vi "G_code_interpriter.vi"() -> ()   [LabVIEW 2019]
uses:
  <vilib>/Instr/_visa.llb/VISA Configure Serial Port (Instr).vi
panel:
  in  "Выберите COM порт, к которому\nподключено устрйоство":refnum<visa-resource-name>
  in  "stop":bool
  in  "Выбор режима":enum32{"Автоматический режи", "Ручной режим"}(tab)
  out "Номер выполняемой\nстроки":i32
  out "Сейчас выполняется":string[](array[string])
  in  "Исполняемый код":string="%\nG00 X50 Y50 Z10\nG01 X80 Y80\nG03 X120 Y120\nG04 P500\nG03 X50 Y50\nG00 X50 Y50 Z50\nM30\n"
  in  "Автоматический режим старт":bool
  in  "Вверх 2":bool
  in  "?":T1(radio)
  in  "Вниз 2":bool
  in  "Ручной режим старт":bool
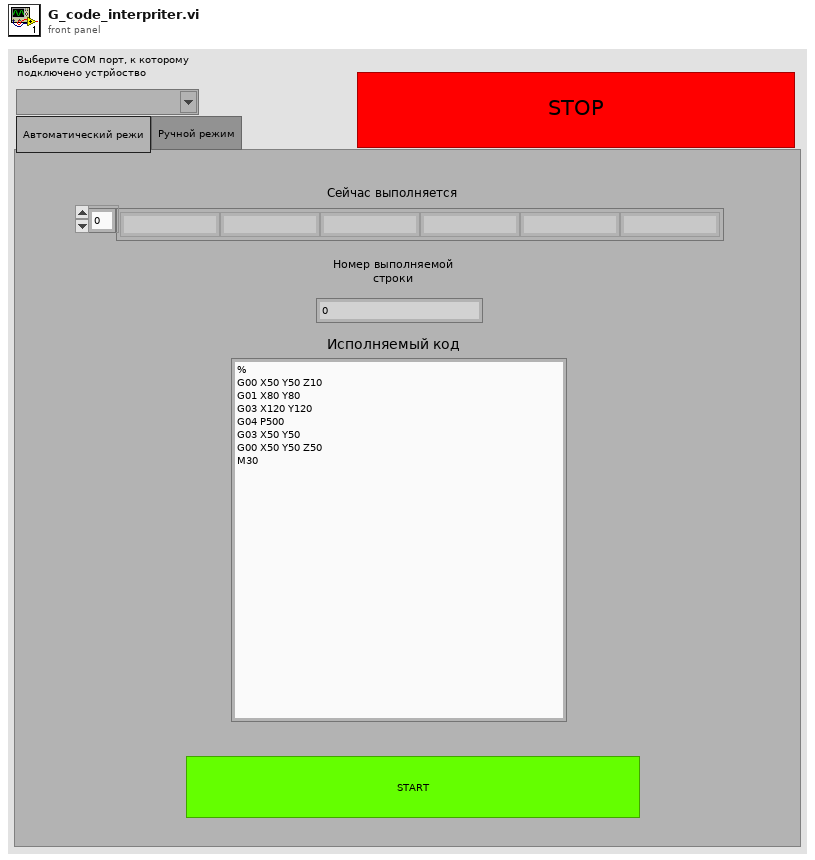
[diagram p1: front panel]
types:
  T1 = enum32{"Перемещение по координате X, 1мм", "Перемещение по координате Y, 1мм", "Перемещение по координате Z, 1мм", "Вращение схвата"}
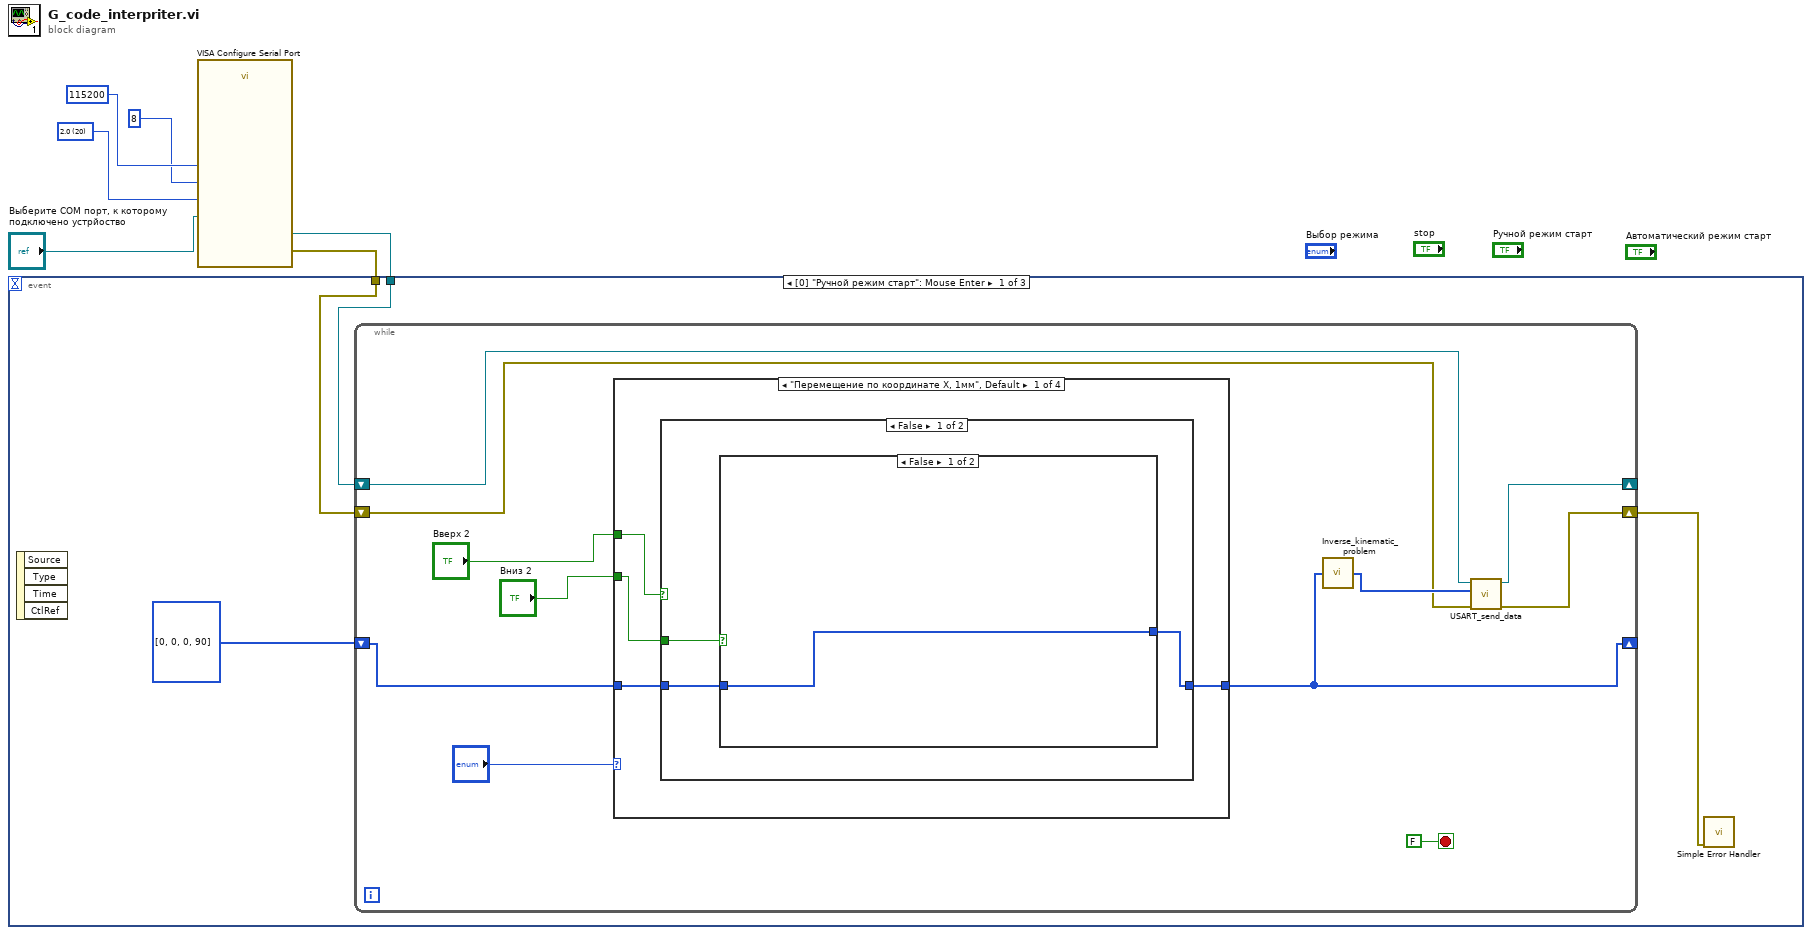
[diagram p0: block diagram]
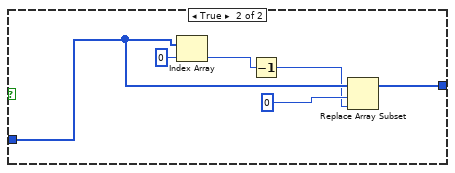
[diagram p2: hidden frame]
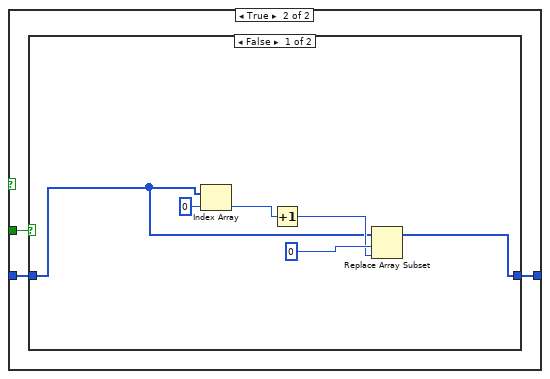
[diagram p3: hidden frame]
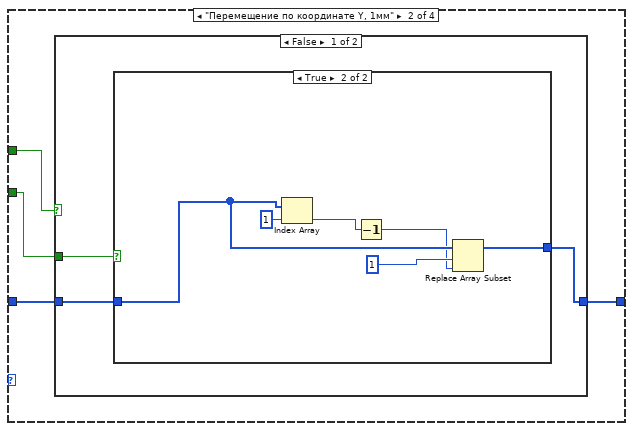
[diagram p5: hidden frame]
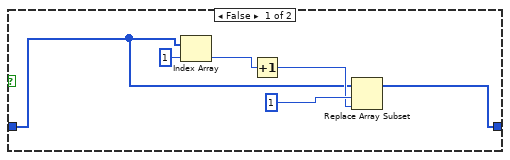
[diagram p8: hidden frame]
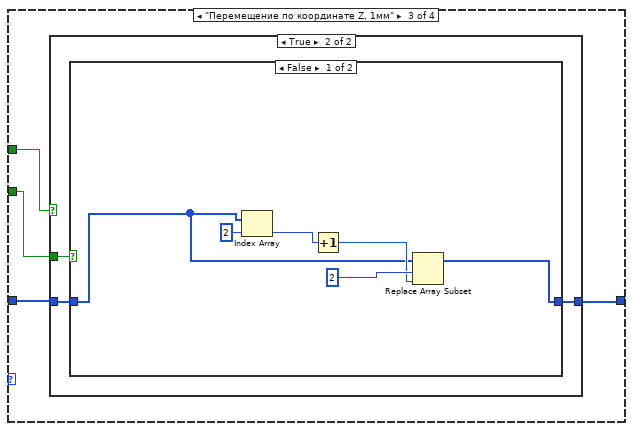
[diagram p9: hidden frame]
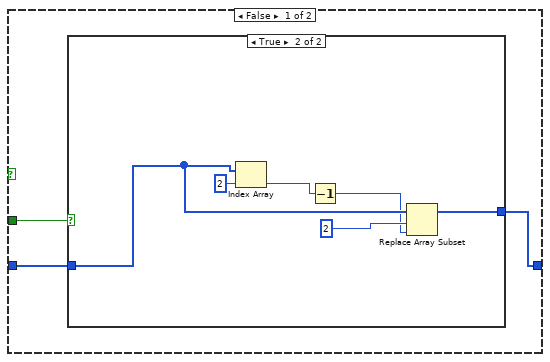
[diagram p10: hidden frame]
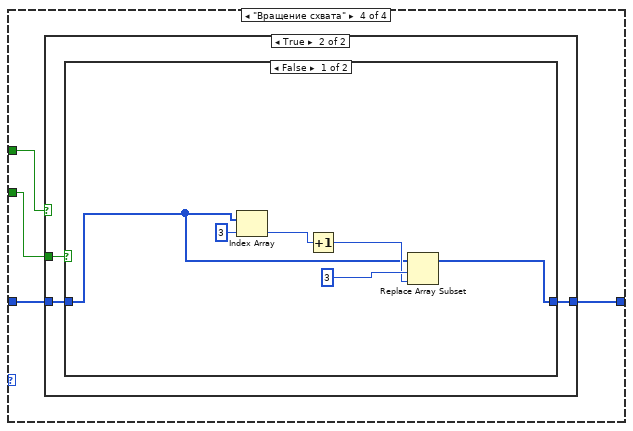
[diagram p13: hidden frame]
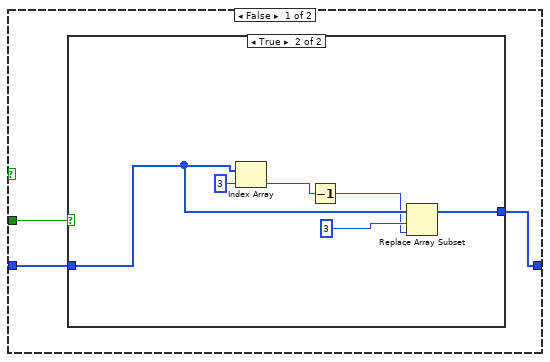
[diagram p14: hidden frame]
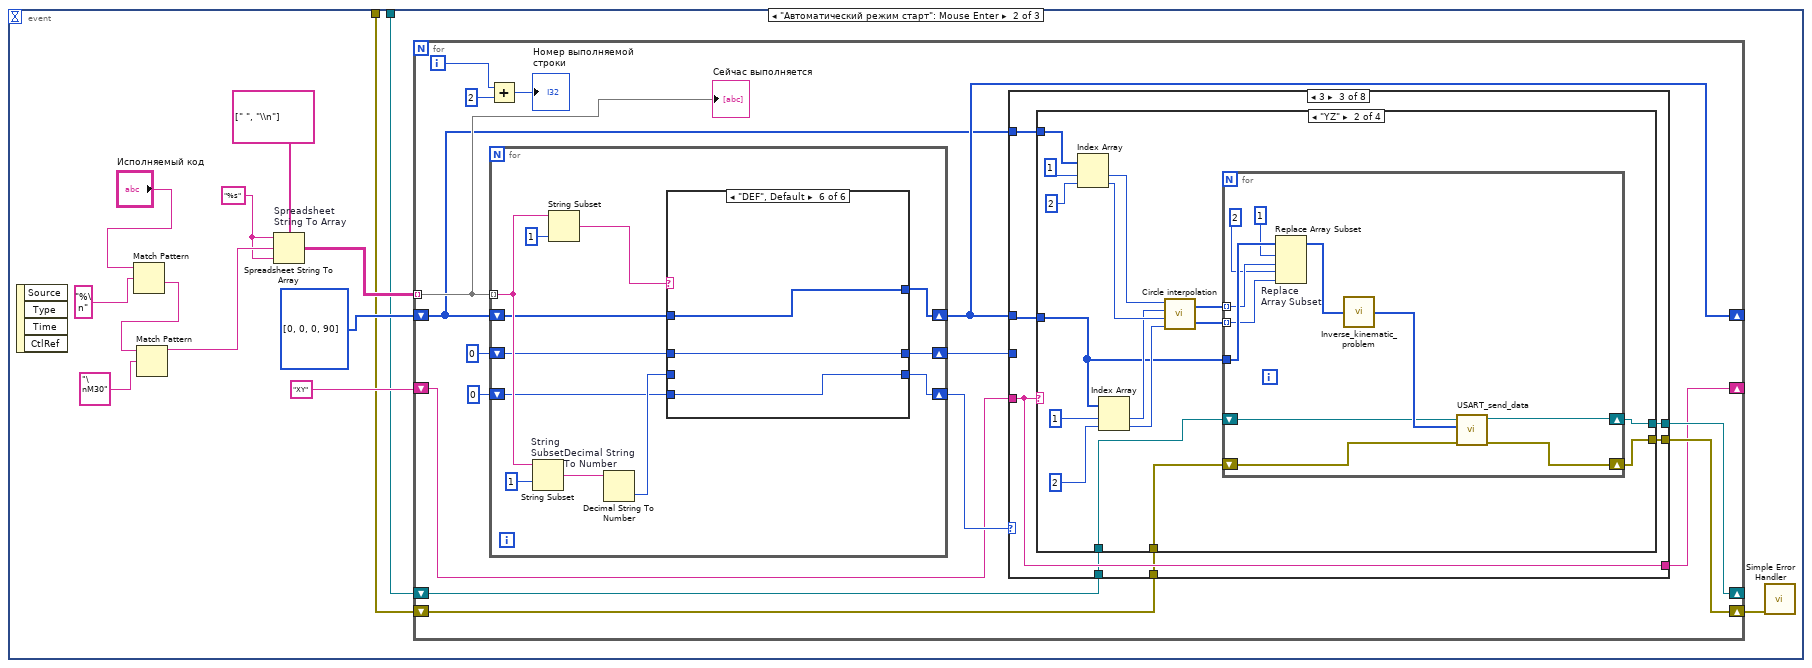
[diagram p17: hidden frame]
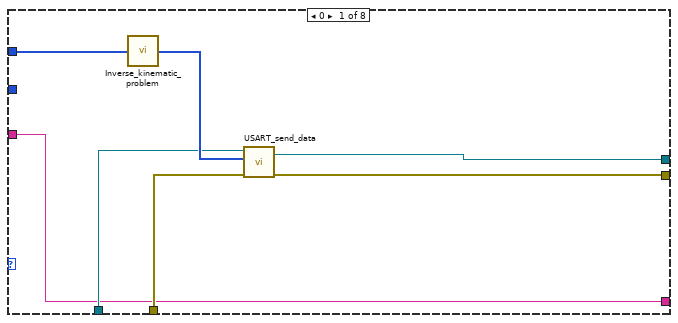
[diagram p18: hidden frame]
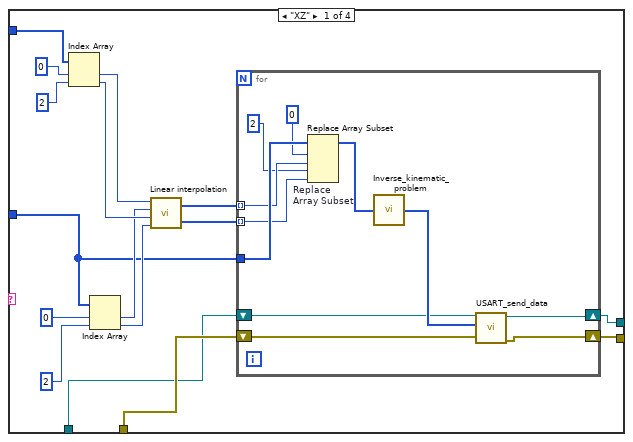
[diagram p20: hidden frame]
diagram:
  w3 = u16 20 items=["1.0"=10, "1.5"=15, "2.0"=20] ("stop bits (10: 1 bit)")
  n1 = call-poly "VISA Configure Serial Port"("VISA resource name"="Выберите COM порт, к которому\nподключено устрйоство", "baud rate (9600)"=u32 115200, "data bits (8)"=u16 8, "stop bits (10: 1 bit)"=w3) -> ("VISA resource name out"=w1:refnum<visa-resource-name>, "error out"=w2:errorcluster)  [unwired: 10 in]
  n2 = event shown="[0] \"Ручной режим старт\": Mouse Enter" {
    selector: _ -> [_ _ _]
    dyn-events: _ -> [_ _ _]
    timeout: _ -> [_ _ _]
    tunnel: w1 -> [w9 w119 _]
    tunnel: w2 -> [w8 w118 _]
    event "Ручной режим старт": Mouse Enter {
      n3 = event-data() -> ()  [unwired: 1 in, 4 out]
      n4 = while {
        shift-right: [w11] -> _
        shift-left: i32[] [0, 0, 0, 90] -> [w18]
        shift-right: [w13] -> _
        shift-left: w9 -> [w15]
        shift-right: [w12] -> w7
        shift-left: w8 -> [w14]
        stop <- FALSE stop-if-true
        n5 = case shown="\"Перемещение по координате X, 1мм\", Default" "?" {
          tunnel: w18 -> [w23 w49 w73 w97]
          tunnel: "Вверх 2" -> [w25 w48 w71 w95]
          tunnel: "Вниз 2" -> [w24 w47 w70 w94]
          tunnel: [w22 w46 w72 w96] -> w11
          frame "Перемещение по координате X, 1мм", Default {
            n6 = case shown="False" w25 {
              tunnel: w24 -> [w28 w38]
              tunnel: w23 -> [w27 w37]
              tunnel: [w26 w36] -> w22
              frame False {
                n7 = case shown="False" w28 {
                  tunnel: w27 -> [w29 w33]
                  tunnel: [w29 w30] -> w26
                  frame False {
                  }
                  frame True {
                    n8 = Index Array(array=w33, index=0) -> (element=w31:i32)
                    n9 = Decrement(x=w31) -> (x-1=w32:i32)
                    n10 = Replace Array Subset(array=w33, new element=w32, index=0) -> (w30:i32[])
                  }
                }
              }
              frame True {
                n11 = case shown="False" w38 {
                  tunnel: w37 -> [w40 w45]
                  tunnel: [w39 w45] -> w36
                  frame False {
                    n12 = Index Array(array=w40, index=0) -> (element=w43:i32)
                    n13 = Increment(x=w43) -> (x+1=w41:i32)
                    n14 = Replace Array Subset(array=w40, new element=w41, index=0) -> (w39:i32[])
                  }
                  frame True {
                  }
                }
              }
            }
          }
          frame "Перемещение по координате Y, 1мм" {
            n15 = case shown="False" w48 {
              tunnel: w47 -> [w52 w62]
              tunnel: w49 -> [w51 w61]
              tunnel: [w50 w60] -> w46
              frame False {
                n16 = case shown="True" w52 {
                  tunnel: w51 -> [w53 w57]
                  tunnel: [w53 w54] -> w50
                  frame False {
                  }
                  frame True {
                    n17 = Index Array(array=w57, index=1) -> (element=w55:i32)
                    n18 = Decrement(x=w55) -> (x-1=w56:i32)
                    n19 = Replace Array Subset(array=w57, new element=w56, index=1) -> (w54:i32[])
                  }
                }
              }
              frame True {
                n20 = case shown="True" w62 {
                  tunnel: w61 -> [w64 w69]
                  tunnel: [w63 w69] -> w60
                  frame False {
                    n21 = Index Array(array=w64, index=1) -> (element=w67:i32)
                    n22 = Increment(x=w67) -> (x+1=w65:i32)
                    n23 = Replace Array Subset(array=w64, new element=w65, index=1) -> (w63:i32[])
                  }
                  frame True {
                  }
                }
              }
            }
          }
          frame "Перемещение по координате Z, 1мм" {
            n24 = case shown="True" w71 {
              tunnel: w70 -> [w76 w86]
              tunnel: w73 -> [w75 w85]
              tunnel: [w74 w84] -> w72
              frame False {
                n25 = case shown="True" w76 {
                  tunnel: w75 -> [w77 w81]
                  tunnel: [w77 w78] -> w74
                  frame False {
                  }
                  frame True {
                    n26 = Index Array(array=w81, index=2) -> (element=w79:i32)
                    n27 = Decrement(x=w79) -> (x-1=w80:i32)
                    n28 = Replace Array Subset(array=w81, new element=w80, index=2) -> (w78:i32[])
                  }
                }
              }
              frame True {
                n29 = case shown="False" w86 {
                  tunnel: w85 -> [w88 w93]
                  tunnel: [w87 w93] -> w84
                  frame False {
                    n30 = Index Array(array=w88, index=2) -> (element=w91:i32)
                    n31 = Increment(x=w91) -> (x+1=w89:i32)
                    n32 = Replace Array Subset(array=w88, new element=w89, index=2) -> (w87:i32[])
                  }
                  frame True {
                  }
                }
              }
            }
          }
          frame "Вращение схвата" {
            n33 = case shown="True" w95 {
              tunnel: w94 -> [w100 w110]
              tunnel: w97 -> [w99 w109]
              tunnel: [w98 w108] -> w96
              frame False {
                n34 = case shown="True" w100 {
                  tunnel: w99 -> [w101 w105]
                  tunnel: [w101 w102] -> w98
                  frame False {
                  }
                  frame True {
                    n35 = Index Array(array=w105, index=3) -> (element=w103:i32)
                    n36 = Decrement(x=w103) -> (x-1=w104:i32)
                    n37 = Replace Array Subset(array=w105, new element=w104, index=3) -> (w102:i32[])
                  }
                }
              }
              frame True {
                n38 = case shown="False" w110 {
                  tunnel: w109 -> [w112 w117]
                  tunnel: [w111 w117] -> w108
                  frame False {
                    n39 = Index Array(array=w112, index=3) -> (element=w115:i32)
                    n40 = Increment(x=w115) -> (x+1=w113:i32)
                    n41 = Replace Array Subset(array=w112, new element=w113, index=3) -> (w111:i32[])
                  }
                  frame True {
                  }
                }
              }
            }
          }
        }
        n42 = call "Inverse_kinematic_problem.vi"("Необходимое\nположение\nсхвата"=w11) -> ("Coords"=w16:u32[])
        n43 = call "USART_send_data.vi"("error in"=w14, "Coordinates"=w16, "VISA resource name in"=w15) -> ("error out"=w12:errorcluster, "VISA resource name out"=w13:refnum<visa-resource-name>)  [unwired: 7 in]
      }
      n44 = call <vilib>:"Simple Error Handler.vi"("error in (no error)"=w7) -> ()  [unwired: 4 in, 5 out]
    }
    event "Автоматический режим старт": Mouse Enter {
      w121 = "%s" ("format string")
      n45 = event-data() -> ()  [unwired: 1 in, 4 out]
      n46 = Match Pattern(string="Исполняемый код", regular expression="%\n") -> (after substring=w126:string)  [unwired: 1 in, 3 out]
      n47 = Match Pattern(string=w126, regular expression="\nM30") -> (before substring=w127:string)  [unwired: 1 in, 3 out]
      n48 = Spreadsheet String To Array "Spreadsheet\nString To Array"(delimiter (Tab)=string[] [" ", "\\n"], format string=w121, spreadsheet string=w127, array type (2D Dbl)=w121) -> (array=w128:string[][])
      n49 = for {
        tunnel: w128 -> [w146] mode=indexing
        shift-right: [w141] -> _
        shift-left: i32[] [0, 0, 0, 90] -> [w140]
        shift-right: [w139] -> w129
        shift-left: w118 -> [w138]
        shift-right: [w134] -> _
        shift-left: "XY" -> [w137]
        shift-right: [w135] -> _
        shift-left: w119 -> [w136]
        i -> [w133]
        n50 = Add(x=w133, y=2) -> (x+y=→"Номер выполняемой\nстроки":i32)
        n51 = for {
          tunnel: w146 -> [w366] mode=indexing
          shift-right: [w357] -> w143
          shift-left: 0 -> [w360]
          shift-right: [w358] -> w141
          shift-left: w140 -> [w359]
          shift-right: [w356] -> w142
          shift-left: 0 -> [w355]
          n52 = String Subset "String\nSubset"(string=w366, offset (0)=1) -> (substring=w362:string)  [unwired: 1 in]
          n53 = String Subset(string=w366, length (rest)=1 ("length (rest)")) -> (substring=w363:string)  [unwired: 1 in]
          n54 = Decimal String To Number "Decimal String\nTo Number"(string=w362) -> (number=w361:i32)  [unwired: 2 in, 1 out]
          n55 = case shown="\"DEF\", Default" w363 {
            tunnel: w361 -> [w369 w373 w379 w385 w388 _]
            tunnel: [w369 w375 w381 w387 w389 w393] -> w357
            tunnel: w360 -> [_ w375 w381 w387 w389 w393]
            tunnel: w359 -> [w368 w374 w378 w384 w390 w392]
            tunnel: [w368 w371 w377 w383 w390 w392] -> w358
            tunnel: [w367 w370 w376 w382 w388 w391] -> w356
            tunnel: w355 -> [w367 w370 w376 w382 _ w391]
            frame "G" {
            }
            frame "X" {
              n56 = Replace Array Subset(array=w374, new element=w373, index=0) -> (w371:i32[])
            }
            frame "Y" {
              n57 = Replace Array Subset(array=w378, new element=w379, index=1) -> (w377:i32[])
            }
            frame "Z" {
              n58 = Replace Array Subset "Replace Array Subset"(array=w384, new element=w385, index=2) -> (w383:i32[])
            }
            frame "P" {
            }
            frame "DEF", Default {
            }
          }
        }
        n59 = case shown="3" w143 {
          tunnel: w142 -> [_ _ _ w337 _ _ _ _]
          tunnel: w141 -> [w153 w159 w249 _ _ _ _ _]
          tunnel: w140 -> [_ w160 w248 _ _ _ _ _]
          tunnel: w136 -> [w151 w157 w246 w335 w339 w342 w345 w348]
          tunnel: w138 -> [w150 w158 w247 w336 w340 w343 w346 w349]
          tunnel: [w149 w156 w244 w336 w340 w343 w346 w349] -> w139
          tunnel: w137 -> [w147 w154 w250 w334 _ _ _ w347]
          tunnel: [w148 w155 w245 w335 w339 w342 w345 w348] -> w135
          tunnel: [w147 w154 w250 w334 "XY" "XZ" "YZ" w347] -> w134
          frame 0 {
            n60 = call "Inverse_kinematic_problem.vi"("Необходимое\nположение\nсхвата"=w153) -> ("Coords"=w152:u32[])
            n61 = call "USART_send_data.vi"("error in"=w150, "Coordinates"=w152, "VISA resource name in"=w151) -> ("error out"=w149:errorcluster, "VISA resource name out"=w148:refnum<visa-resource-name>)  [unwired: 7 in]
          }
          frame 1 {
            n62 = case shown="\"DEF\", Default" w154 {
              tunnel: w160 -> [w166 w193 w220 _]
              tunnel: w159 -> [w165 w192 w218 _]
              tunnel: w158 -> [w164 w191 w219 w243]
              tunnel: w157 -> [w162 w189 w216 w242]
              tunnel: [w163 w190 w217 w243] -> w156
              tunnel: [w161 w188 w215 w242] -> w155
              frame "XZ" {
                n63 = Index Array(array=w166, index #1=0 ("index"), index #2=2 ("index")) -> (element #1=w172:i32, element #2=w171:i32)
                n64 = Index Array(array=w165, index #1=0 ("index"), index #2=2 ("index")) -> (element #1=w170:i32, element #2=w169:i32)
                n65 = call "Linear interpolation.vi"("Yf"=w169, "Y0"=w171, "Xf"=w170, "X0"=w172) -> ("Y array"=w167:i32[], "X array"=w168:i32[])
                n66 = for {
                  tunnel: w168 -> [w186] mode=indexing
                  tunnel: w167 -> [w185] mode=indexing
                  tunnel: w165 -> [w187]
                  shift-right: [w179] -> w163
                  shift-left: w164 -> [w180]
                  shift-right: [w177] -> w161
                  shift-left: w162 -> [w178]
                  n67 = Replace Array Subset "Replace\nArray Subset"(array=w187, new element #1=w186, index #1=0 ("index"), new element #2=w185, index #2=2 ("index")) -> (w181:i32[])
                  n68 = call "Inverse_kinematic_problem.vi"("Необходимое\nположение\nсхвата"=w181) -> ("Coords"=w182:u32[])
                  n69 = call "USART_send_data.vi"("error in"=w180, "Coordinates"=w182, "VISA resource name in"=w178) -> ("error out"=w179:errorcluster, "VISA resource name out"=w177:refnum<visa-resource-name>)  [unwired: 7 in]
                }
              }
              frame "XY" {
                n70 = Index Array(array=w193, index #1=0 ("index"), index #2=1 ("index")) -> (element #1=w199:i32, element #2=w198:i32)
                n71 = Index Array(array=w192, index #1=0 ("index"), index #2=1 ("index")) -> (element #1=w197:i32, element #2=w196:i32)
                n72 = call "Linear interpolation.vi"("Yf"=w196, "Y0"=w198, "Xf"=w197, "X0"=w199) -> ("Y array"=w194:i32[], "X array"=w195:i32[])
                n73 = for {
                  tunnel: w195 -> [w213] mode=indexing
                  tunnel: w194 -> [w212] mode=indexing
                  tunnel: w192 -> [w214]
                  shift-right: [w206] -> w190
                  shift-left: w191 -> [w207]
                  shift-right: [w204] -> w188
                  shift-left: w189 -> [w205]
                  n74 = Replace Array Subset "Replace\nArray Subset"(array=w214, new element #1=w213, index #1=0 ("index"), new element #2=w212, index #2=1 ("index")) -> (w208:i32[])
                  n75 = call "Inverse_kinematic_problem.vi"("Необходимое\nположение\nсхвата"=w208) -> ("Coords"=w209:u32[])
                  n76 = call "USART_send_data.vi"("error in"=w207, "Coordinates"=w209, "VISA resource name in"=w205) -> ("error out"=w206:errorcluster, "VISA resource name out"=w204:refnum<visa-resource-name>)  [unwired: 7 in]
                }
              }
              frame "YZ" {
                n77 = Index Array(array=w220, index #1=1 ("index"), index #2=2 ("index")) -> (element #1=w226:i32, element #2=w225:i32)
                n78 = Index Array(array=w218, index #1=1 ("index"), index #2=2 ("index")) -> (element #1=w224:i32, element #2=w223:i32)
                n79 = call "Linear interpolation.vi"("Yf"=w223, "Y0"=w225, "Xf"=w224, "X0"=w226) -> ("Y array"=w221:i32[], "X array"=w222:i32[])
                n80 = for {
                  tunnel: w222 -> [w240] mode=indexing
                  tunnel: w221 -> [w239] mode=indexing
                  tunnel: w218 -> [w241]
                  shift-right: [w233] -> w217
                  shift-left: w219 -> [w234]
                  shift-right: [w231] -> w215
                  shift-left: w216 -> [w232]
                  n81 = Replace Array Subset "Replace\nArray Subset"(array=w241, new element #1=w240, index #1=1 ("index"), new element #2=w239, index #2=2 ("index")) -> (w235:i32[])
                  n82 = call "Inverse_kinematic_problem.vi"("Необходимое\nположение\nсхвата"=w235) -> ("Coords"=w236:u32[])
                  n83 = call "USART_send_data.vi"("error in"=w234, "Coordinates"=w236, "VISA resource name in"=w232) -> ("error out"=w233:errorcluster, "VISA resource name out"=w231:refnum<visa-resource-name>)  [unwired: 7 in]
                }
              }
              frame "DEF", Default {
              }
            }
          }
          frame 3 {
            n84 = case shown="\"YZ\"" w250 {
              tunnel: w249 -> [w255 w283 _ w312]
              tunnel: w248 -> [w256 w282 _ w311]
              tunnel: w247 -> [w253 w280 w305 w310]
              tunnel: w246 -> [w254 w281 w306 w309]
              tunnel: [w252 w279 w306 w308] -> w245
              tunnel: [w251 w278 w305 w307] -> w244
              frame "XZ" {
                n85 = Index Array(array=w256, index #1=0 ("index"), index #2=2 ("index")) -> (element #1=w261:i32, element #2=w263:i32)
                n86 = Index Array(array=w255, index #1=0 ("index"), index #2=2 ("index")) -> (element #1=w262:i32, element #2=w264:i32)
                n87 = call "Circle interpolation.vi"("Yf"=w264, "Y0"=w263, "Xf"=w262, "X0"=w261) -> ("Y array"=w265:i32[], "X array"=w266:i32[])
                n88 = for {
                  tunnel: w266 -> [w276] mode=indexing
                  tunnel: w265 -> [w275] mode=indexing
                  tunnel: w255 -> [w277]
                  shift-right: [w269] -> w251
                  shift-left: w253 -> [w270]
                  shift-right: [w267] -> w252
                  shift-left: w254 -> [w268]
                  n89 = Replace Array Subset "Replace\nArray Subset"(array=w277, new element #1=w276, index #1=0 ("index"), new element #2=w275, index #2=2 ("index")) -> (w271:i32[])
                  n90 = call "Inverse_kinematic_problem.vi"("Необходимое\nположение\nсхвата"=w271) -> ("Coords"=w272:u32[])
                  n91 = call "USART_send_data.vi"("error in"=w270, "Coordinates"=w272, "VISA resource name in"=w268) -> ("error out"=w269:errorcluster, "VISA resource name out"=w267:refnum<visa-resource-name>)  [unwired: 7 in]
                }
              }
              frame "YZ" {
                n92 = Index Array(array=w282, index #1=1 ("index"), index #2=2 ("index")) -> (element #1=w288:i32, element #2=w290:i32)
                n93 = Index Array(array=w283, index #1=1 ("index"), index #2=2 ("index")) -> (element #1=w289:i32, element #2=w291:i32)
                n94 = call "Circle interpolation.vi"("Yf"=w291, "Y0"=w290, "Xf"=w289, "X0"=w288) -> ("Y array"=w292:i32[], "X array"=w293:i32[])
                n95 = for {
                  tunnel: w293 -> [w303] mode=indexing
                  tunnel: w292 -> [w302] mode=indexing
                  tunnel: w283 -> [w304]
                  shift-right: [w296] -> w278
                  shift-left: w280 -> [w297]
                  shift-right: [w294] -> w279
                  shift-left: w281 -> [w295]
                  n96 = Replace Array Subset "Replace\nArray Subset"(array=w304, new element #1=w303, index #1=1 ("index"), new element #2=w302, index #2=2 ("index")) -> (w298:i32[])
                  n97 = call "Inverse_kinematic_problem.vi"("Необходимое\nположение\nсхвата"=w298) -> ("Coords"=w299:u32[])
                  n98 = call "USART_send_data.vi"("error in"=w297, "Coordinates"=w299, "VISA resource name in"=w295) -> ("error out"=w296:errorcluster, "VISA resource name out"=w294:refnum<visa-resource-name>)  [unwired: 7 in]
                }
              }
              frame "DEF", Default {
              }
              frame "XY" {
                n99 = Index Array(array=w311, index #1=0 ("index"), index #2=1 ("index")) -> (element #1=w317:i32, element #2=w319:i32)
                n100 = Index Array(array=w312, index #1=0 ("index"), index #2=1 ("index")) -> (element #1=w318:i32, element #2=w320:i32)
                n101 = call "Circle interpolation.vi"("Yf"=w320, "Y0"=w319, "Xf"=w318, "X0"=w317) -> ("Y array"=w321:i32[], "X array"=w322:i32[])
                n102 = for {
                  tunnel: w322 -> [w332] mode=indexing
                  tunnel: w321 -> [w331] mode=indexing
                  tunnel: w312 -> [w333]
                  shift-right: [w325] -> w307
                  shift-left: w310 -> [w326]
                  shift-right: [w323] -> w308
                  shift-left: w309 -> [w324]
                  n103 = Replace Array Subset "Replace\nArray Subset"(array=w333, new element #1=w332, index #1=0 ("index"), new element #2=w331, index #2=1 ("index")) -> (w327:i32[])
                  n104 = call "Inverse_kinematic_problem.vi"("Необходимое\nположение\nсхвата"=w327) -> ("Coords"=w328:u32[])
                  n105 = call "USART_send_data.vi"("error in"=w326, "Coordinates"=w328, "VISA resource name in"=w324) -> ("error out"=w325:errorcluster, "VISA resource name out"=w323:refnum<visa-resource-name>)  [unwired: 7 in]
                }
              }
            }
          }
          frame 4 {
            n106 = Wait (ms)(milliseconds to wait=w337) -> ()  [unwired: 1 out]
          }
          frame 17 {
          }
          frame 18 {
          }
          frame 19 {
          }
          frame 999, Default {
            n107 = Two Button Dialog(message="Неподдерживаемый G-code.\nПродолжить выполненеие программы?", 1:"Остановить программу" ("F button name (\"Cancel\")"), 2:"Продолжить" ("T button name (\"OK\")")) -> (T button?=w350:bool)
            n108 = Not(x=w350) -> (.not. x?=w351:bool)
            n109 = Stop(stop? (T)=w351) -> ()
          }
        }
        "Сейчас выполняется" <- w146
      }
      n110 = call <vilib>:"Simple Error Handler.vi"("error in (no error)"=w129) -> ()  [unwired: 4 in, 5 out]
    }
    event "stop": Mouse Enter {
      n111 = event-data() -> ()  [unwired: 1 in, 4 out]
      n112 = One Button Dialog(message="Выполнение программы остановлено.\nДля запуска выберите режим и нажимите СТАРТ") -> ()  [unwired: 1 in, 1 out]
    }
  }
